vi "test_fpga_scanClocks.vi"() -> ()   [LabVIEW 2016]
uses:
  <vilib>/Platform/TimedLoop/XDataNode/XDataNode.xnode
  <vilib>/Platform/TimedLoop/XDataNode/nitl_modes.ctl
  <vilib>/Platform/TimedLoop/XDataNode/XDNodeRunTimeDep.lvlib
  <vilib>/Platform/TimedLoop/XDataNode/wakeup.ctl
  <vilib>/Platform/TimedLoop/XDataNode/timing_clust.ctl
panel:
  out "moveIndices":cluster{"index":u16, "next":u16}
  out "clocks":T1
  out "fastIndices":cluster{"index":u16, "next":u16}
  in  "resetClocks":bool
  in  "moveRates":T2
  in  "scanRates":T3={"outputRate"=50, "fastDecFactor"=0, "outWaveSizeFast"=0, "pplUpsampling"=0, "numLines"=0}
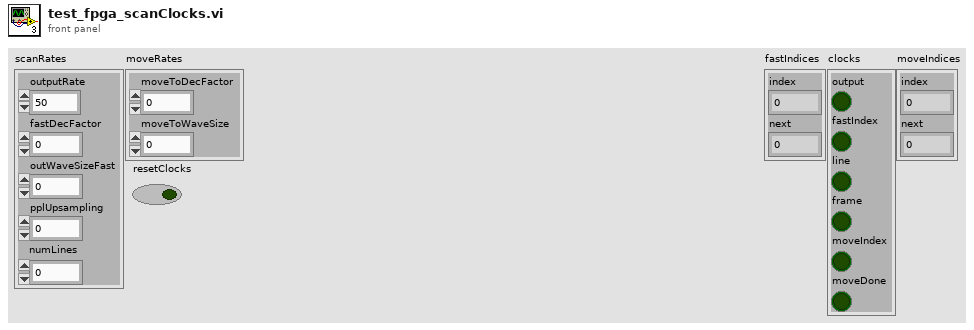
[diagram p1: front panel]
types:
  T1 = cluster{"output":bool, "fastIndex":bool, "line":bool, "frame":bool, "moveIndex":bool, "moveDone":bool}
  T2 = cluster{"moveToDecFactor":u16, "moveToWaveSize":u16}
  T3 = cluster{"outputRate":u16, "fastDecFactor":u16, "outWaveSizeFast":u16, "pplUpsampling":u16, "numLines":u16}
  T4 = typedef "XDNodeRunTimeDep.lvlib/timing_clust.ctl" = cluster{"Expected End [f-1]":u64, "Actual End [f-1]":u64, "Finished Late? [f-1]":bool, "Expected End [i-1]":u64, "Actual End [i-1]":u64, "Finished Late? [i-1]":bool, "Expected Start [i]":u64, "Actual Start [i]":u64, "Expected Start [f]":u64, "Actual Start [f]":u64, "Source Name":string, "Structure Name":string, "Period":i64, "Deadline":i64, "Offset":i64, "Start":i64, "Priority":i32, "Timeout":i32, "Mode":T5, "Wakeup Reason":T6, "Error":errorcluster, "Source Type":string, "Secondary Source Type":string, "Global End Time":u64, "Global Start Time":u64, "Frame Duration":u64, "Iteration Duration":u64, "Assigned CPU":i32, "I/O Scan Engine Mode":u32}
  T5 = typedef "XDNodeRunTimeDep.lvlib/nitl_modes.ctl" = enum32{"No Change", "Process missed periods, maintain original phase", "Discard missed periods, maintain original phase", "Process missed periods, ignore original phase", "Discard missed periods, ignore original phase"}
  T6 = typedef "XDNodeRunTimeDep.lvlib/wakeup.ctl" = enum32{"Normal", "Aborted", "Asynchronous wakeup", "Timing source error", "Timed loop error", "Timeout"}
  T7 = cluster{"output":bool, "fastIndex":bool, "line":bool, "frame":bool, "moveIndex":bool, "moveDone":bool, "pixel":bool}
  T8 = cluster{"index":u16, "next":u16, "blanking":u32, "blankingNext":u32}
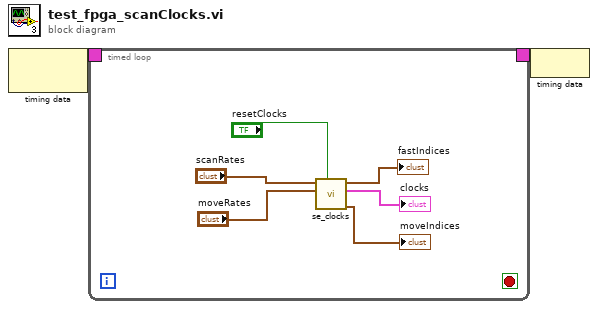
[diagram p0: block diagram]
diagram:
  n1 = node-c288() -> (w2:T4)  [unwired: 1 in]
  n2 = timed-loop {
    timing: w2 -> [_]
    timing-out: [_] -> w1
    stop <- _ stop-if-true
    n3 = call "se_clocks.vi"("se.p.resetClocks"="resetClocks", "moveRates"="moveRates", "se.p.clocks"="scanRates") -> ("moveIndices"=→"moveIndices":cluster{"index":u16, "next":u16}, "clocks"=→"clocks":T7, "fastIndices"=→"fastIndices":T8)  [unwired: 5 in, 1 out]
  }
  n4 = node-c288(w1) -> ()
